vi "edit-data.vi"(10 "Hardware Resources in":T1={"DAQmx Channel 1"="", "DAQmx Channel 2"="", "DAQmx Channel 3"="", "Channel 1 Name"="", "Channel 2 Name"="", "Channel 3 Name"="", "Input Config Channel 1"=-1, "Input Config Channel 2"=-1, "Input Config Channel 3"=-1, "Offset Channel 1"=0.0, "Offset Channel 2"=0.0, "Offset Channel 3"=0.0, "Scale Channel 1"=0.0, "Scale Channel 2"=0.0, "Scale Channel 3"=0.0, "DAQmx Counter Channel"="", "Counter Name"="", "Sample time"=0, "Samples per second"=0.0, "Sample mode"=0, "Samples per channel"=0, "DAQmx AI Task"="", "DAQmx Counter Task"=""} {"Input Config Channel 3" items=["Default"=-1, "RSE"=10083, "NRSE"=10078, "Differential"=10106, "Pseudodifferential"=12529]; "Input Config Channel 2" items=["Default"=-1, "RSE"=10083, "NRSE"=10078, "Differential"=10106, "Pseudodifferential"=12529]; "Input Config Channel 1" items=["Default"=-1, "RSE"=10083, "NRSE"=10078, "Differential"=10106, "Pseudodifferential"=12529]; "Sample mode" items=["Hardware Timed Single Point"=12522, "Finite Samples"=10178, "Continuous Samples"=10123]}, 11 "data":waveform(dbl)[](array[waveform])) -> (3 "Array of Waveform":waveform(dbl)[](array[waveform]))   [LabVIEW 2018, in "Acquisition.lvlib"]
uses:
  Acquisition.lvlib
  Hardware Configuration.ctl
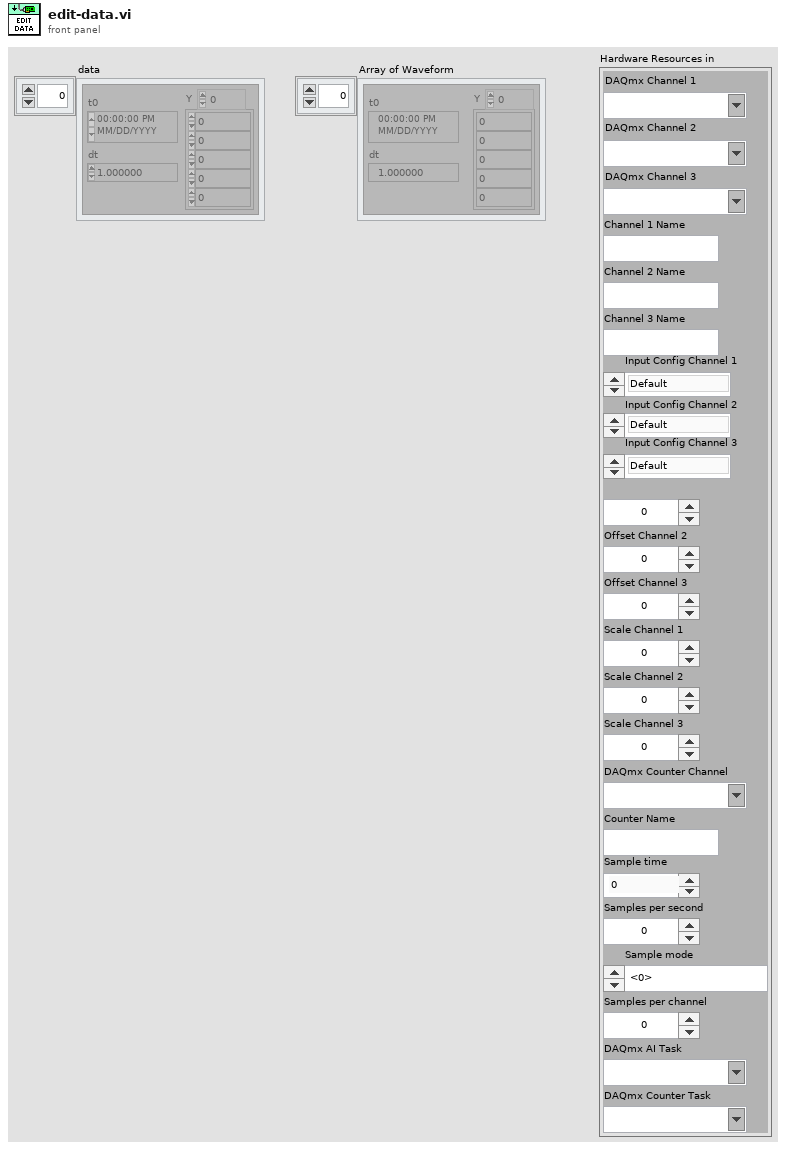
[diagram p1: front panel]
types:
  T1 = typedef "Acquisition.lvlib/Hardware Configuration.ctl" = cluster{"DAQmx Channel 1":tag, "DAQmx Channel 2":tag, "DAQmx Channel 3":tag, "Channel 1 Name":string, "Channel 2 Name":string, "Channel 3 Name":string, "Input Config Channel 1":i32, "Input Config Channel 2":i32, "Input Config Channel 3":i32, "Offset Channel 1":dbl, "Offset Channel 2":dbl, "Offset Channel 3":dbl, "Scale Channel 1":dbl, "Scale Channel 2":dbl, "Scale Channel 3":dbl, "DAQmx Counter Channel":tag, "Counter Name":string, "Sample time":u32, "Samples per second":dbl, "Sample mode":u16, "Samples per channel":i32, "DAQmx AI Task":refnum<k21>, "DAQmx Counter Task":refnum<k21>}
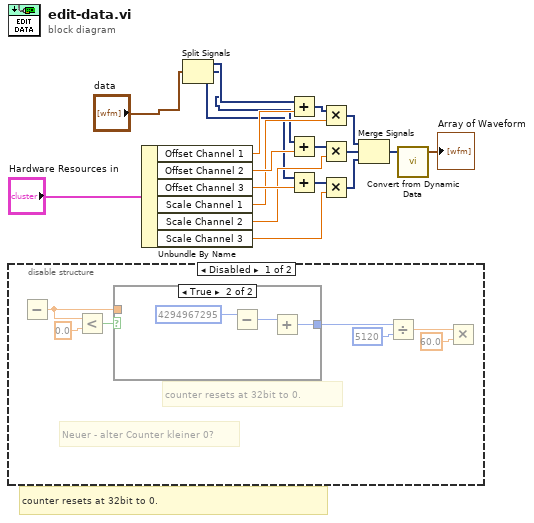
[diagram p0: block diagram]
diagram:
  # "counter resets at 32bit to 0."
  n1 = disable-structure shown="Disabled" {
    frame Disabled {
      # "Neuer - alter Counter kleiner 0?"
      # "counter resets at 32bit to 0."
      n2 = Subtract() -> (x-y=w20:dbl)  [unwired: 2 in]
      n3 = Less?(x=w20, y=0.0) -> (x < y?=w22:bool)
      n4 = case shown="True" w22 {
        tunnel: [_ w27] -> w26
        tunnel: w20 -> [_ _]
        frame False {
        }
        frame True {
          n5 = Subtract(x=u32 4294967295 ("y")) -> (x-y=w28:u32)  [unwired: 1 in]
          n6 = Add(x=w28) -> (x+y=w27:u32)  [unwired: 1 in]
        }
      }
      n7 = Divide(x=w26, y=u32 5120) -> (x/y=w24:dbl)
      n8 = Multiply(x=w24, y=60.0) -> ()  [unwired: 1 out]
    }
    frame Enabled {
    }
  }
  n9 = Unbundle By Name("Hardware Resources in") -> ("Offset Channel 1"=w14:dbl, "Offset Channel 2"=w16:dbl, "Offset Channel 3"=w18:dbl, "Scale Channel 1"=w15:dbl, "Scale Channel 2"=w17:dbl, "Scale Channel 3"=w19:dbl)
  n10 = Split Signals("data") -> (w3:dynamicdata, w2:dynamicdata, w1:dynamicdata)  [unwired: 3 in]
  n11 = Add(x=w3, y=w14) -> (x+y=w5:dynamicdata)
  n12 = Add(x=w2, y=w16) -> (x+y=w6:dynamicdata)
  n13 = Add(x=w1, y=w18) -> (x+y=w7:dynamicdata)
  n14 = Multiply(x=w5, y=w15) -> (x*y=w8:dynamicdata)
  n15 = Multiply(x=w6, y=w17) -> (x*y=w9:dynamicdata)
  n16 = Multiply(x=w7, y=w19) -> (x*y=w10:dynamicdata)
  n17 = Merge Signals(w8, w9, w10) -> (w11:dynamicdata)
  n18 = call "Convert from Dynamic Data"("Dynamic Data Type"=w11) -> ("Array of Waveform"=→"Array of Waveform":waveform(dbl)[])  [unwired: 3 in]
